vi "Clear Variable Forcing.vi"(6 "error in (no error)":errorcluster, 9 "target address (localhost)":string="localhost") -> (0 "error out":errorcluster)   [LabVIEW 2017]
doc: "Unforces all currently forced I/O variables and I/O aliases on the target."
uses:
  <resource>/objmgr/ni.var.rc
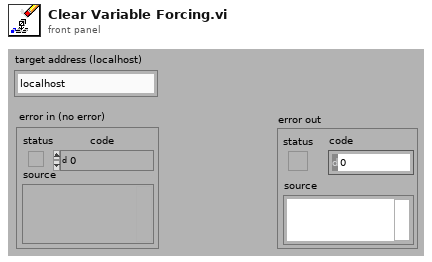
[diagram p1: front panel]
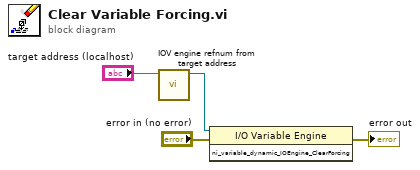
[diagram p0: block diagram]
diagram:
  n1 = call <vilib>:"IOV engine refnum from target address.vi"("target address"="target address (localhost)") -> ("reference out"=w3:refnum<k21>)  [unwired: 10 in]
  n2 = invoke class="I/O Variable Engine" method="ni_variable_dynamic_IOEngine_ClearForcing"(reference=w3, error in="error in (no error)") -> (error out=→"error out":errorcluster)  [unwired: 1 in, 2 out]
